vi "Tetra_Rev.vi"(0 "COMPORT":refnum<visa-resource-name>="COM4", 11 "error in (no error)":errorcluster, 13 "Open Ser(t)":bool, 14 "Close Ser(t)":bool) -> (1 "pmic_rev":string="#PMIC_Rev: 1.1", 2 "Success":bool, 3 "rev":string="#SW_Version: 02002008 Rev 2.2.8\n#SW_GitHash: 1A16B09D\n#SW_Date: 20221212\n#FW_Version: 02020105 Rev 2.2.1 HW Rev 5\n#FW_GitHash: A587BC9D\n#FW_Date: 20221101\r\n", 4 "comport":refnum<visa-resource-name>="COM4", 15 "error out":errorcluster)   [LabVIEW 2018]
doc: "This example performs writes and reads on a serial port, as directed by the user. You can press the Write and Read buttons, and change the Read Count, while the example is running.\n\nThe parameters set for the serial port must match the parameters of the connected instrument or device. In this example, the Read Count parameter specifies the number of bytes that the serial port reads. If there were more bytes at the port than the specified number, those bytes would not be read. If there were less bytes at the port than the specified number, you would receive a timeout error.\n\nThis example expands upon the flow control options for XON and XOFF, allowing the user to choose those control characters. Also, the user can enable or disable a termination character. Some devices require a termination character in order to identify the end of command strings. Some devices send a termination character to signify the end of data to be read. This example shows how you can end the Read operation once a termination character is detected in the buffer and/or append a termination character at the end of the Write data."
panel:
  # "0xA is equivalent to a '\\n' character, which is a line feed."
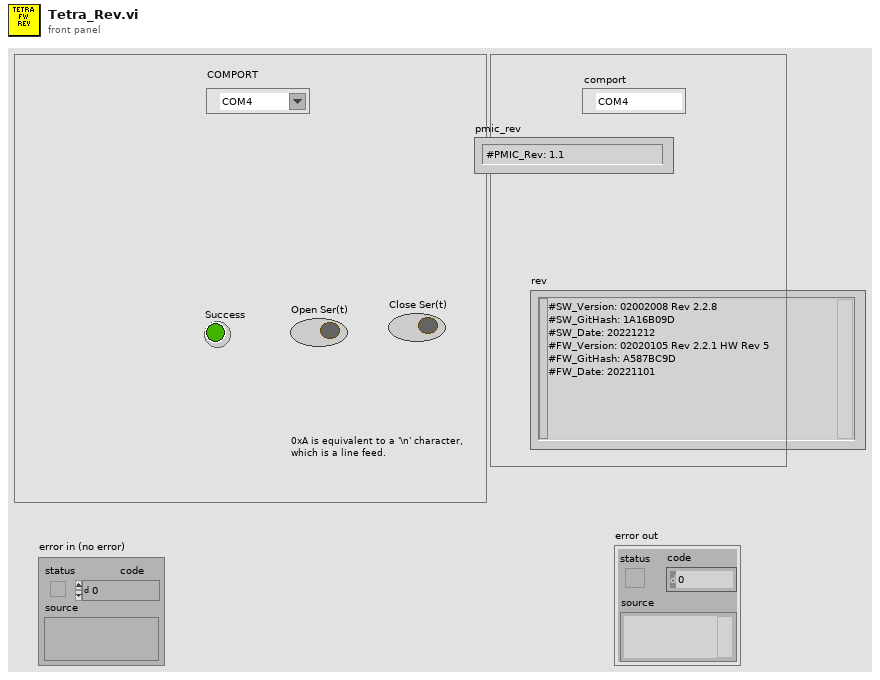
[diagram p1: front panel]
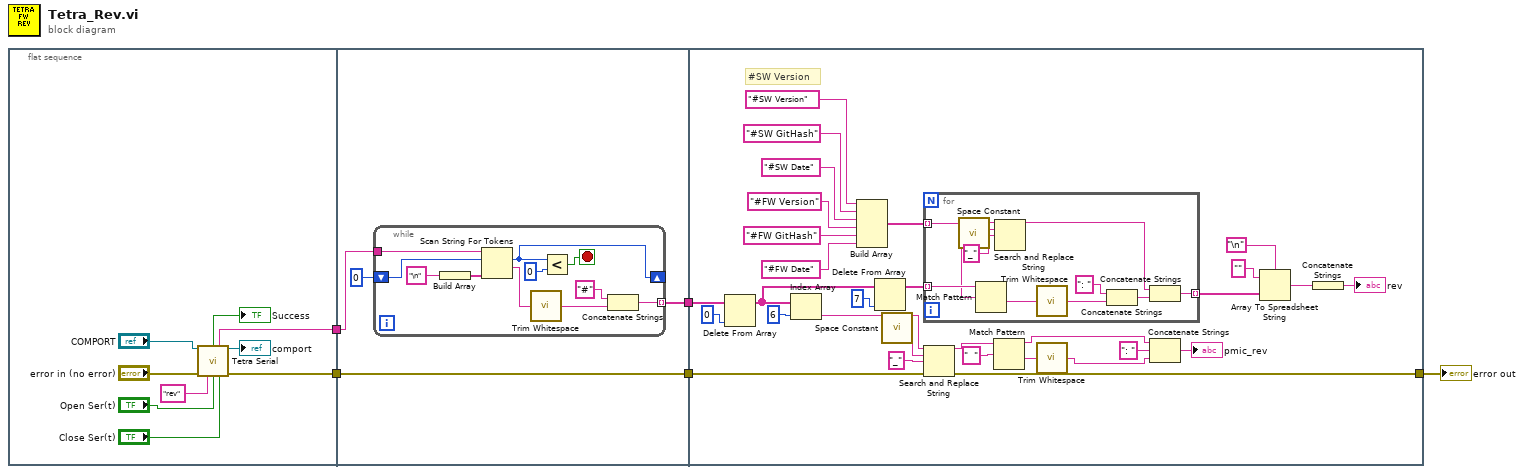
[diagram p0: block diagram]
diagram:
  n1 = flat-sequence {
    tunnel: [w7] -> w5
    tunnel: [w6] -> w3
    tunnel: w5 -> [w17]
    tunnel: [w18] -> w4
    tunnel: w3 -> [w15]
    tunnel: [w15] -> w2
    tunnel: w4 -> [w35]
    tunnel: w2 -> [w31]
    tunnel: [w30] -> w1
    frame #0 {
      n2 = call "Tetra Serial.vi"("COMPORT"="COMPORT", "error in (no error)"="error in (no error)", "Command"="rev", "Open Ser(t)"="Open Ser(t)", "Close Ser(t)"="Close Ser(t)") -> ("Success"=→"Success":bool, "output"=w7:string, "comport"=→"comport":refnum<visa-resource-name>, "error out"=w6:errorcluster)  [unwired: 7 in]
    }
    frame #1 {
      n3 = while {
        tunnel: [w20] -> w18 mode=indexing
        shift-right: [w27] -> _
        shift-left: 0 ("offset past token") -> [w26]
        tunnel: w17 -> [w24]
        stop <- w28 stop-if-true
        n4 = Build Array("\n") -> (w25:string[])
        n5 = Scan String For Tokens(6:w25, 8:w26, 9:w24) -> (1:w21:string, 2:w27:i32)  [unwired: 3 in, 2 out]
        n6 = call <vilib>:"Trim Whitespace.vi"("string"=w21) -> ("trimmed string"=w19:string)  [unwired: 1 in]
        n7 = Less?(x=w27, y=0) -> (x < y?=w28:bool)
        n8 = Concatenate Strings("#" ("string"), w19) -> (w20:string)
      }
    }
    frame #2 {
      # "#SW Version"
      n9 = Delete From Array(array=w35, index=0) -> (array with subset deleted=w56:string[])  [unwired: 1 in, 1 out]
      n10 = Index Array(array=w56, index=6) -> (element=w49:string)
      n11 = Build Array("#SW Version", "#SW GitHash" ("element"), "#SW Date" ("element"), "#FW Version", "#FW GitHash" ("element"), "#FW Date" ("element")) -> (w58:string[])
      n12 = Delete From Array(array=w56, index=7) -> (array with subset deleted=w57:string[])  [unwired: 1 in, 1 out]
      n13 = call <vilib>:"Space Constant.vi"() -> ("String"=w50:string)
      n14 = for {
        tunnel: w57 -> [w69] mode=indexing
        tunnel: w58 -> [w65] mode=indexing
        tunnel: [w60] -> w59 mode=indexing
        n15 = call <vilib>:"Space Constant.vi"() -> ("String"=w64:string)
        n16 = Match Pattern(string=w69, regular expression=w65) -> (after substring=w66:string)  [unwired: 1 in, 3 out]
        n17 = Search and Replace String(input string=w65, search string=w64, replace string="_" ("replace string (\"\")")) -> (result string=w62:string)  [unwired: 5 in, 3 out]
        n18 = call <vilib>:"Trim Whitespace.vi"("string"=w66) -> ("trimmed string"=w67:string)  [unwired: 1 in]
        n19 = Concatenate Strings(": " ("string"), w67) -> (w61:string)
        n20 = Concatenate Strings(w62, w61) -> (w60:string)
      }
      n21 = Search and Replace String(input string=w49, search string=w50, replace string="_" ("replace string (\"\")"), error in=w31) -> (result string=w51:string, error out=w30:errorcluster)  [unwired: 4 in, 2 out]
      n22 = Match Pattern(string=w51, regular expression="  ") -> (before substring=w53:string, after substring=w52:string)  [unwired: 1 in, 2 out]
      n23 = call <vilib>:"Trim Whitespace.vi"("string"=w52) -> ("trimmed string"=w54:string)  [unwired: 1 in]
      n24 = Concatenate Strings(w53, ": " ("string"), w54) -> (→"pmic_rev":string)
      n25 = Array To Spreadsheet String(delimiter (Tab)="\n", array=w59, 3:"" ("format string")) -> (spreadsheet string=w47:string)
      n26 = Concatenate Strings(w47) -> (→"rev":string)
    }
  }
  "error out" <- w1
